vi "SMAC.vi"(5 "write buffer":string, 7 "VISA resource name":refnum<visa-resource-name>) -> ()   [LabVIEW 2023]
uses:
  <vilib>/Instr/_visa.llb/VISA Configure Serial Port (Instr).vi
panel:
  out "error out":errorcluster
  out "read buffer":string
  out "return count":u32
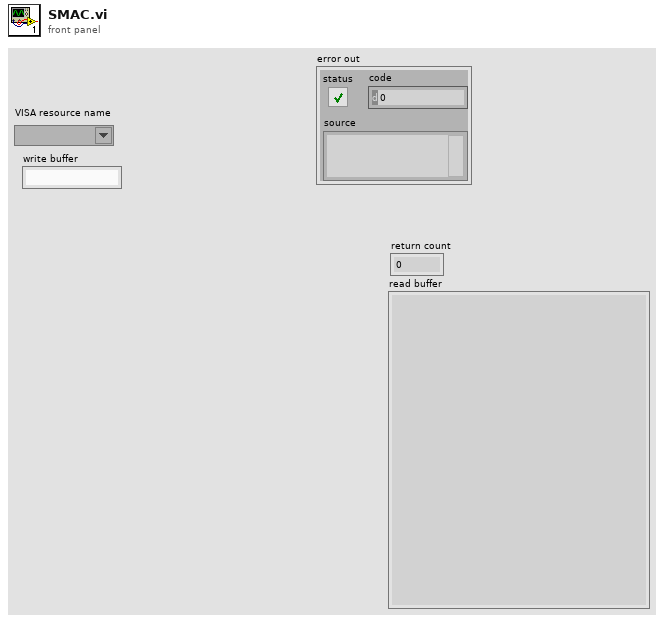
[diagram p1: front panel]
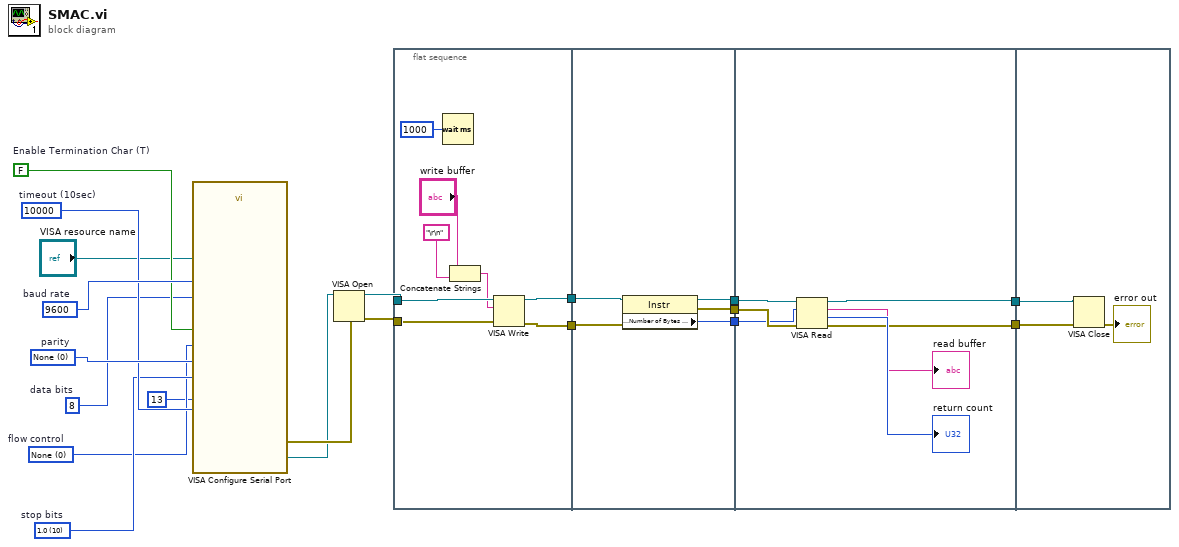
[diagram p0: block diagram]
diagram:
  w20 = u32 9600  # baud rate
  w15 = u16 0 items=["None"=0, "XON/XOFF"=1, "RTS/CTS"=2, "DTR/DSR"=4]  # flow control
  w16 = u16 10 items=["1.0"=10, "1.5"=15, "2.0"=20]  # stop bits
  w19 = u16 0 items=["None", "Odd", "Even", "Mark", "Space"]  # parity
  w14 = u16 8  # data bits
  w17 = FALSE  # Enable Termination Char (T)
  w18 = u32 10000  # timeout (10sec)
  n1 = call-poly "VISA Configure Serial Port"("VISA resource name"="VISA resource name", "timeout (10sec)"=w18, "termination char\n(0xA = '\\n' = LF)"=u8 13 ("termination char\n(0xA = '\\n' = LF)"), "Enable Termination\nChar (T)"=w17, "baud rate (9600)"=w20, "data bits (8)"=w14, "parity (0:none)"=w19, "stop bits (10: 1 bit)"=w16, "flow control (0:none)"=w15) -> ("VISA resource name out"=w1:refnum<visa-resource-name>, "error out"=w2:errorcluster)  [unwired: 5 in]
  n2 = VISA Open(error in (no error)=w2, VISA resource name=w1) -> (VISA resource name=w10:refnum<visa-resource-name>, error out=w11:errorcluster)  [unwired: 3 in]
  n3 = flat-sequence {
    tunnel: [w26] -> w9
    tunnel: [w25] -> w7
    tunnel: w11 -> [w28]
    tunnel: w10 -> [w27]
    tunnel: w9 -> [w30]
    tunnel: [w31] -> w8
    tunnel: w7 -> [w33]
    tunnel: [w32] -> w6
    tunnel: [w29] -> w3
    tunnel: w8 -> [w40]
    tunnel: w6 -> [w39]
    tunnel: [w36] -> w5
    tunnel: [w35] -> w4
    tunnel: w3 -> [w34]
    tunnel: w5 -> [w43]
    tunnel: w4 -> [w42]
    frame #0 {
      n4 = Wait (ms)(milliseconds to wait=u32 1000) -> ()  [unwired: 1 out]
      n5 = Concatenate Strings("write buffer", "\r\n" ("string")) -> (w21:string)
      n6 = VISA Write(VISA resource name=w27, write buffer=w21, error in (no error)=w28) -> (VISA resource name out=w25:refnum<visa-resource-name>, error out=w26:errorcluster)  [unwired: 1 out]
    }
    frame #1 {
      n7 = property class="Instr"(reference=w33, error in=w30) -> (reference out=w32:refnum<visa-resource-name>, error out=w31:errorcluster, "Serial Settings:Number of Bytes at Serial Port"=w29:u32)
    }
    frame #2 {
      n8 = VISA Read(VISA resource name=w39, byte count=w34, error in (no error)=w40) -> (VISA resource name out=w36:refnum<visa-resource-name>, read buffer=→"read buffer":string, return count=→"return count":u32, error out=w35:errorcluster)
    }
    frame #3 {
      n9 = VISA Close(VISA resource name=w43, error in (no error)=w42) -> (error out=→"error out":errorcluster)
    }
  }
